vi "Einheit Name from Index.vi"(11 "EinheitIndex":T1) -> (3 "EinheitName":string)   [LabVIEW 2020, in "Linearisierung v2.lvlib" / "SpanEinstellungen.lvlib"]
uses:
  SpanEinstellungen.lvlib
  Einheit.ctl
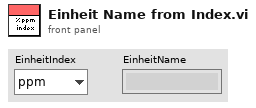
[diagram p1: front panel]
types:
  T1 = typedef "Linearisierung v2.lvlib/SpanEinstellungen.lvlib/Einheit.ctl" = enum16{"ppm", "%"}
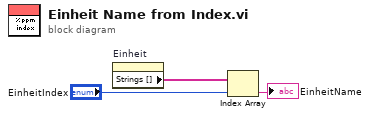
[diagram p0: block diagram]
diagram:
  n1 = property on="Einheit" class="Enum (strikt)"() -> ("Strings []"=w3:string[])  [unwired: 2 in, 2 out]
  n2 = Index Array(array=w3, index="EinheitIndex") -> (element=→"EinheitName":string)
